vi "Termocupla y LM35 con Arduino.vi"() -> ()   [LabVIEW 2026]
uses:
  <vilib>/MakerHub/LINX/Public/Peripherals/Analog/Analog Read 1 Chan.vi
  <vilib>/MakerHub/LINX/Public/Peripherals/Analog/Analog Read N Chans.vi
  <vilib>/MakerHub/LINX/Private/Local IO/LinxAnalogRead.vi
  <vilib>/MakerHub/LINX/Public/Utilities/Check Channel.vi
  <vilib>/MakerHub/LINX/Public/Utilities/Open Serial.vi
  <vilib>/MakerHub/LINX/Private/Utilties/Generate Error.vi
  <vilib>/MakerHub/LINX/LMH-LINX.lvlib
panel:
  out "Numeric 2":dbl
  out "Numeric":dbl
  in  "Canal Termocupla":u8
  out "Termocupla K":dbl(slide) scale=0.0..100.0
  out "LM35":dbl(slide) scale=0.0..100.0
  in  "stop":bool
  in  "Canal LM35":u8
  in  "Baud Rate Override":u32
  in  "Serial Port":refnum<visa-resource-name>="N/A"
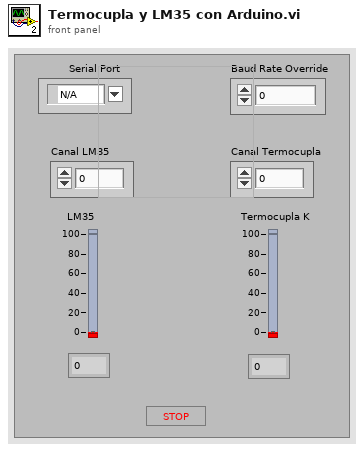
[diagram p1: front panel]
types:
  T1 = typedef "LMH-LINX.lvlib/LINX Ref.ctl" = cluster{"IO":T2, "Interface":T3, "LINX Device Config":T4}
  T2 = typedef "LMH-LINX.lvlib/Platform.ctl" = enum16{"Remote", "Local"}
  T3 = typedef "LMH-LINX.lvlib/Interface.ctl" = enum16{"Serial", "TCP"}
  T4 = typedef "LMH-LINX.lvlib/Device.lvlib/LINX Device Config.ctl" = cluster{"Interface":T3, "COM Port":refnum<visa-resource-name>, "TCP Configuration":T5, "Device Family":u8, "Device ID":u8, "Device Name":string, "TCP Ref":refnum<k5>, "Channels":T6}
  T5 = typedef "LMH-LINX.lvlib/Device.lvlib/TCP Config.ctl" = cluster{"IP Address":string, "Port":u16}
  T6 = typedef "LMH-LINX.lvlib/Channels.ctl" = cluster{"DI":u8[], "DO":u8[], "AI":u8[], "AO":u8[], "PWM":u8[], "QE":u8[], "UART":u8[], "I2C 2":u8[], "SPI":u8[], "CAN":u8[], "Servo":u8[], "AI Ref (V)":dbl, "AI Resolution (Bits)":u8, "AO Ref (V)":dbl, "AO Resolution (Bits)":u8}
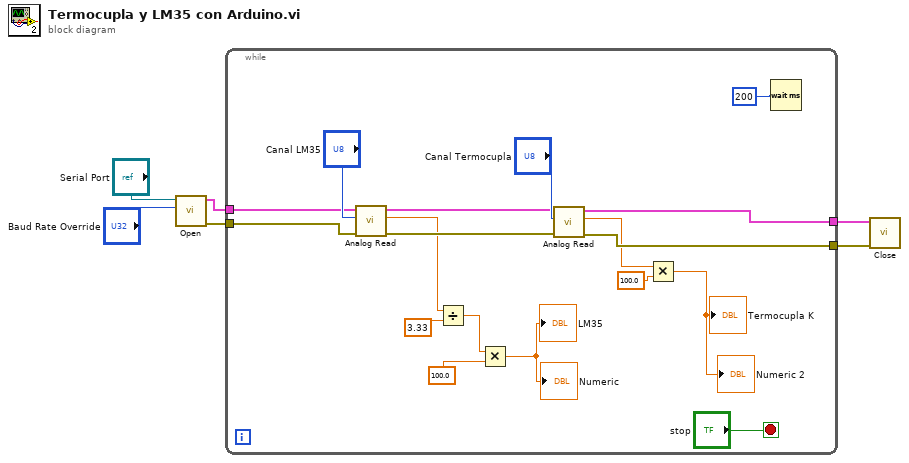
[diagram p0: block diagram]
diagram:
  n1 = call-poly <vilib>:"Open.vi"("Baud Rate Override"="Baud Rate Override", "Serial Port"="Serial Port") -> ("Error Out"=w1:errorcluster, "LINX Resource"=w4:T1)  [unwired: 7 in, 1 out]
  n2 = while {
    tunnel: w4 -> [w23]
    tunnel: [w19] -> w3
    tunnel: [w18] -> w2
    tunnel: w1 -> [w16]
    stop <- "stop" stop-if-true
    n3 = call-poly <vilib>:"Analog Read.vi"("Error In"=w16, "Analog Channel"="Canal LM35", "LINX Resource"=w23) -> ("Error Out"=w17:errorcluster, "Voltage"=w14:dbl, "LINX Resource"=w20:T1)  [unwired: 5 in, 1 out]
    n4 = Divide(x=w14, y=3.33) -> (x/y=w13:dbl)
    n5 = Multiply(x=w13, y=100.0) -> (x*y=→"LM35" →"Numeric":dbl)
    n6 = call-poly <vilib>:"Analog Read.vi"("Error In"=w17, "Analog Channel"="Canal Termocupla", "LINX Resource"=w20) -> ("Error Out"=w18:errorcluster, "Voltage"=w8:dbl, "LINX Resource"=w19:T1)  [unwired: 5 in, 1 out]
    n7 = Multiply(x=w8, y=100.0) -> (x*y=→"Termocupla K" →"Numeric 2":dbl)
    n8 = Wait (ms)(milliseconds to wait=u32 200) -> ()  [unwired: 1 out]
  }
  n9 = call <vilib>:"Close.vi"("Error In"=w2, "LINX Resource"=w3) -> ()  [unwired: 9 in, 1 out]
